vi "initialize.vi"(7 "references":T2, 8 "error in (no error)":errorcluster, 11 "configuration":T1) -> (0 "error out":errorcluster)   [LabVIEW 2015, in "lv-recipe-machine.lvlib"]
uses:
  lv-recipe-machine.lvlib
  _controls/references.ctl
  _controls/input.ctl
  _controls/input_command.ctl
  _controls/output.ctl
  _controls/transition.ctl
  _controls/data.ctl
  _controls/configuration.ctl
  _controls/recipe_data.ctl
  _controls/mode.ctl
  _controls/manual_state.ctl
  _controls/automatic_state.ctl
  _controls/timer.ctl
  _controls/recipe_step.ctl
  _controls/change.ctl
  _controls/status.ctl
  private/_controls/timers.ctl
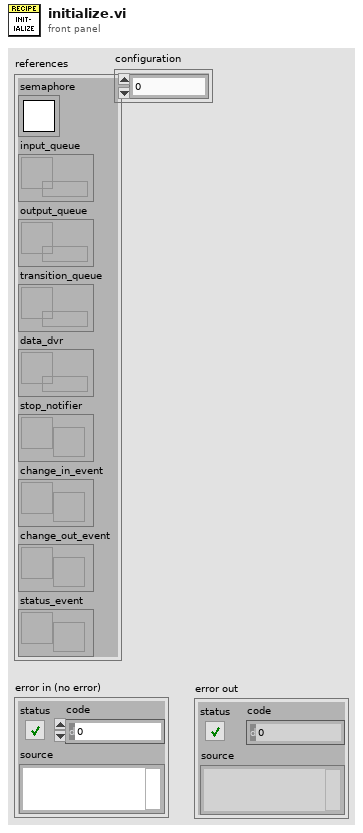
[diagram p1: front panel]
types:
  T1 = typedef "lv-recipe-machine.lvlib/configuration.ctl" = cluster{dbl}
  T2 = typedef "lv-recipe-machine.lvlib/references.ctl" = cluster{"semaphore":T3, "input_queue":refnum<queue>, "output_queue":refnum<queue>, "transition_queue":refnum<queue>, "data_dvr":refnum<data-value>, "stop_notifier":refnum<notifier>, "change_in_event":refnum<user-event>, "change_out_event":refnum<user-event>, "status_event":refnum<user-event>}
  T3 = typedef "Semaphore RefNum" = refnum<k1>
  T4 = typedef "lv-recipe-machine.lvlib/timer.ctl" = cluster{"elapsed_time":dbl, "previous_time":dbl}
  T5 = typedef "lv-recipe-machine.lvlib/timers.ctl" = enum16{"<timers>", "step", "recipe", "<null>"}
  T6 = typedef "lv-recipe-machine.lvlib/data.ctl" = cluster{"configuration":T1, "working":cluster{"recipe_data":T7}}
  T7 = typedef "lv-recipe-machine.lvlib/recipe_data.ctl" = cluster{"mode":T8, "manual_state":T9, "automatic_state":T10, "previous_automatic_state":T10, "error":errorcluster, "timer []":T4[], "manual":cluster{"step_action":string, "data":variant, "actions":variant}, "automatic":cluster{"data":variant, "steps":variant, "criteria":variant, "transition":string, "index":i32, "recipe []":T11[]}}
  T8 = typedef "lv-recipe-machine.lvlib/mode.ctl" = enum16{"<mode>", "manual", "automatic", "<null>"}
  T9 = typedef "lv-recipe-machine.lvlib/manual_state.ctl" = enum16{"<manual_state>", "failed", "action", "running", "idle", "<null>"}
  T10 = typedef "lv-recipe-machine.lvlib/automatic_state.ctl" = enum16{"<automatic_state>", "failed", "idle", "running", "paused", "stopped", "<null>"}
  T11 = typedef "lv-recipe-machine.lvlib/recipe_step.ctl" = cluster{"step":string, "data":variant}
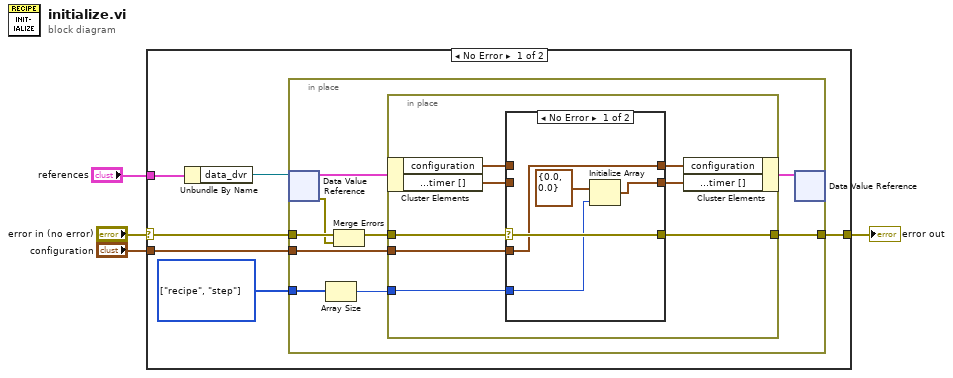
[diagram p0: block diagram]
diagram:
  n1 = case shown="No Error" "error in (no error)" {
    selector: "error in (no error)" -> [w9 w36]
    tunnel: [w6 w36] -> w3
    tunnel: "references" -> [w7 _]
    tunnel: "configuration" -> [w8 _]
    frame No Error {
      w5 = T5[] [enum."recipe", enum."step"] items=["<timers>", "step", "recipe", "<null>"]
      n2 = Unbundle By Name(w7) -> ("data_dvr"=w10:refnum<data-value>)
      n3 = in-place {
        in-place-border: w9 -> [w19]
        in-place-border: w8 -> [w14]
        in-place-border: [w13] -> w6
        in-place-border: w5 -> [w12]
        n4 = in-place-dvr #1(w10) -> (w16:T6, w18:errorcluster)
        n5 = Array Size(array=w12) -> (size(s)=w11:i32)
        n6 = Merge Errors(w19, w18) -> (w17:errorcluster)
        n7 = in-place {
          in-place-border: w17 -> [w23]
          in-place-border: w14 -> [w24]
          in-place-border: [w25] -> w13
          in-place-border: w11 -> [w20]
          n8 = in-place-cluster #2(w16) -> ("configuration"=w27:T1, "working.recipe_data.timer []"=w22:T4[])
          n9 = case shown="No Error" w23 {
            selector: w23 -> [w32 w34]
            tunnel: w24 -> [w31 _]
            tunnel: w27 -> [_ w35]
            tunnel: [w31 w35] -> w26
            tunnel: [w32 w34] -> w25
            tunnel: w22 -> [_ w33]
            tunnel: [w28 w33] -> w21
            tunnel: w20 -> [w29 _]
            frame No Error {
              n10 = Initialize Array(T4 {"elapsed_time"=0.0, "previous_time"=0.0}, w29) -> (w28:T4[])
            }
            frame Error {
            }
          }
          n11 = in-place-cluster #2("configuration"=w26, "working.recipe_data.timer []"=w21) -> (w15:T6)
        }
        n12 = in-place-dvr #1(w15) -> ()  [unwired: 2 out]
      }
    }
    frame Error {
    }
  }
  "error out" <- w3
